vi "UI_main.vi"() -> ()   [LabVIEW 2013]
uses:
  parameter set for calibration.ctl
panel:
  in  "主要控制界面":enum32{"实时图像", "校准图样", "追踪数据", "设置"}(tab)
  out "力值估算":dbl
  out "往返测量":bool
  out "测量中":bool
  out "当前力值计算":dbl
  out "磁铁终点":dbl
  out "磁铁起点":dbl
  out "队列积压数据":u8(slide) scale=0.0..100.0
  out "测量模式":string
  out "文件存放路径":path
  out "测量进度":u8(slide) scale=0.0..100.0
  in  "当前温度":dbl
  in  "磁铁转数":dbl
  in  "磁铁位置":dbl
  in  "焦平面位置":dbl
  out "波形图":dbl[](graph)
  in  "校准磁球编号":dbl
  out "强度图":dbl[][](graph)
  out "D(Y)":dbl
  out "Y方向均值":dbl
  out "D(X)":dbl
  out "X方向均值":dbl
  out "Z_RMSE":dbl
  out "Z方向均值":dbl
  in  "参考磁球编号":enum16{""}(ring)
  in  "测量磁球编号":enum16{""}(ring)
  out "波形图表":dbl(graph)
  out "采样频率":dbl
  out "数据更新频率":dbl
  in  "旋转电机驱动":bool
  in  "步进电机驱动":bool
  in  "CCD相机驱动":bool
  out "单位像素大小":dbl
  in  "ROI size":enum16{"64 ", "128"}(ring)
  in  "显微镜放大倍数":dbl
  out "错误输出":errorcluster
  in  "错误输入（无错误）":errorcluster
  # "实验信息"
  # "数据监测"
  # "磁铁设置"
  # "驱动设置"
  # "ROI设置"
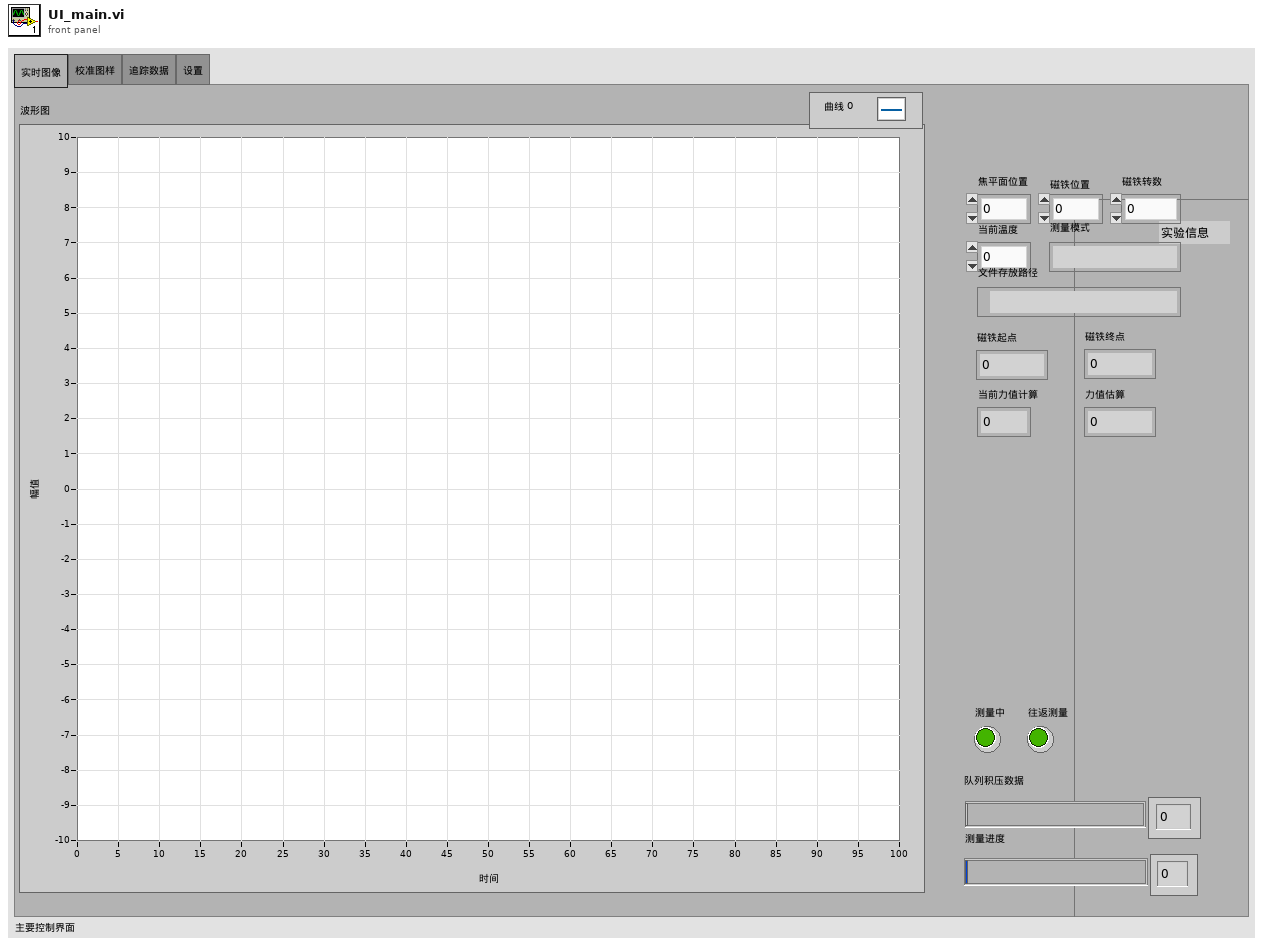
[diagram p1: front panel]
types:
  T1 = typedef "magnet_tweezers_命令.ctl" = enum16{"新建", "打开", "保存", "导出", "退出", "恢复初始设置", "校准", "测量Z值", "WLC", "相机驱动设置", "显微镜设置", "旋转电机设置", "平移电机设置", "保存参数设置", "参考磁球编号", "观测磁球编号", "修改磁铁位置", "修改磁铁转数", "修改当前温度", "修改焦平面位置", "修改磁球编号", "修改ROI大小", "修改显微镜放大倍数"}
  T2 = typedef "前面板命令.ctl" = cluster{"命令":T1, "数据":variant}
  T3 = typedef "tlc_Error Module Command Control.ctl" = enum16{"Initialize", "Handle Errors", "Report Errors"}
  T4 = typedef "parameter set for calibration.ctl" = cluster{"分子长度（bp）":i32, "磁球大小（直径）":dbl[unit], "校准起点":dbl, "校准步长":dbl, "每步采样数（frame）":i32, "首尾去除帧数(frame)":i32, "校准步数":i32, "底面位置":dbl, "R-step":sgl, "R-min":sgl, "R-max":sgl, "num":i32, "x_center":dbl, "y_center":dbl, "磁铁位置":dbl}
  T5 = typedef "parameter set for record.ctl" = cluster{"测量模式":enum16{"force ramp", "force jump", "force clamp"}, "测量起点":dbl, "数据存放路径":path, "加载率":dbl, "初始转数":dbl, "最终转数":dbl, "旋转速度":dbl, "松弛点":dbl, "绷紧点":dbl, "松弛时间":dbl, "绷紧时间":dbl, "步长":dbl, "总步数":dbl, "停留时间":dbl, "测量终点":dbl, "校准完毕？":bool}
  T6 = enum32{"invalid app kind", "Development System", "Run Time System", "Student Edition", "Embedded LabVIEW", "Evaluation", "Custom"}
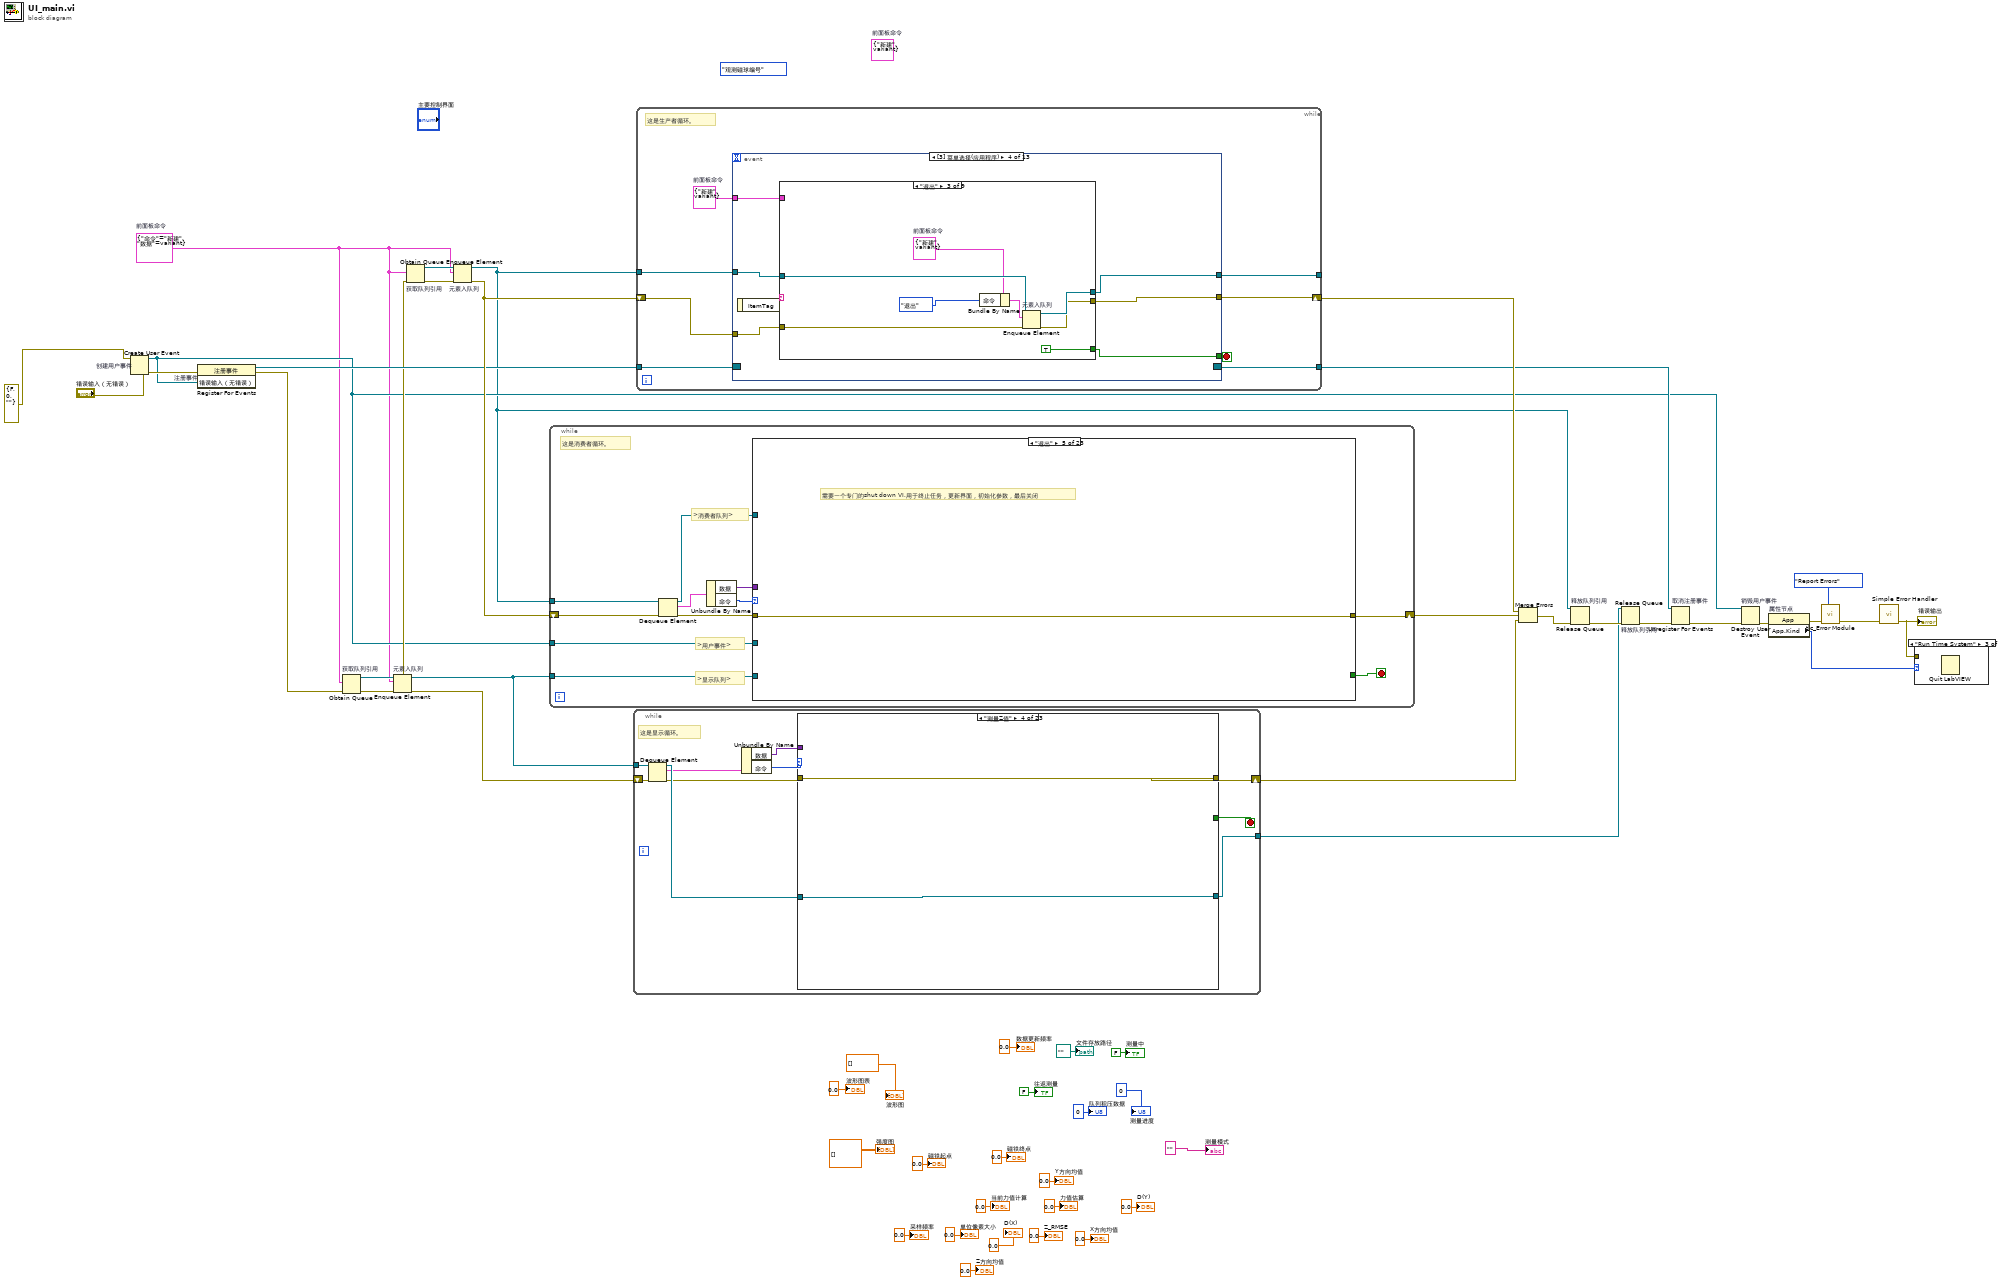
[diagram p0: block diagram]
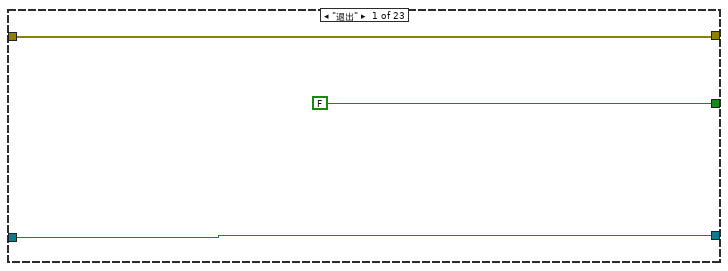
[diagram p8: hidden frame]
diagram:
  (unwired) magnet_tweezers_命令."观测磁球编号" ("命令")
  (unwired) T2 {"命令"=enum."新建", "数据"=variant}  # 前面板命令
  w24 = T2 {"命令"=enum."新建", "数据"=variant}  # 前面板命令
  n1 = Create User Event "创建用户事件"(user event datatype=errorcluster {"status"=FALSE, "code"=0, "source"=""} ("错误输入（无错误）"), error in="错误输入（无错误）") -> (user event=w34:refnum<user-event>, error out=w49:errorcluster)
  n2 = register-events "注册事件"(error in=w49, w34) -> (reference out=w48:refnum<event-registration>, error out=w39:errorcluster)  [unwired: 1 in]
  n3 = Obtain Queue "获取队列引用"(element data type=w24, error in (no error)=w39) -> (queue out=w40:refnum<queue>, error out=w41:errorcluster)  [unwired: 3 in, 1 out]
  n4 = Enqueue Element "元素入队列"(queue=w40, element=w24, error in (no error)=w41) -> (queue out=w33:refnum<queue>, error out=w38:errorcluster)  [unwired: 1 in, 1 out]
  n5 = Obtain Queue "获取队列引用"(element data type=w24, error in (no error)=w38) -> (queue out=w52:refnum<queue>, error out=w51:errorcluster)  [unwired: 3 in, 1 out]
  n6 = Enqueue Element "元素入队列"(queue=w52, element=w24, error in (no error)=w51) -> (queue out=w1:refnum<queue>, error out=w50:errorcluster)  [unwired: 1 in, 1 out]
  n7 = while {
    shift-right: [w53] -> w46
    shift-left: w50 -> [w61]
    tunnel: w1 -> [w63]
    tunnel: w34 -> [w56]
    tunnel: w33 -> [w55]
    stop <- w57 stop-if-true
    # ">显示队列>"
    # ">消费者队列>"
    # ">用户事件>"
    # "这是消费者循环。"
    n8 = Dequeue Element(queue=w63, error in (no error)=w61) -> (queue out=w62:refnum<queue>, element=w60:T2, error out=w58:errorcluster)  [unwired: 1 in, 1 out]
    n9 = Unbundle By Name(w60) -> ("数据"=w54:variant, "命令"=w59:T1)
    n10 = case shown="\"退出\"" w59 {
      tunnel: w62 -> [_ _ _ _ _ _ _ _ _ _ _ _ _ _ _ _ _ _ _ _ _ _ _]
      tunnel: w58 -> [w64 w66 w67 w68 w69 w70 w75 w79 w80 w81 w82 w83 w84 w85 w86 w87 w88 w89 w90 w91 w92 w93 w94]
      tunnel: [FALSE _ _ _ _ _ _ _ _ _ _ _ _ _ _ _ _ _ _ _ _ _ _] -> w57
      tunnel: w56 -> [_ _ _ _ _ _ _ _ _ _ _ _ _ _ _ _ _ _ _ _ _ _ _]
      tunnel: w55 -> [_ _ _ _ _ _ _ _ _ _ _ _ _ _ _ _ _ _ _ _ _ _ _]
      tunnel: w54 -> [_ _ _ _ _ _ w77 _ _ _ _ _ _ _ _ _ _ _ _ _ _ _ _]
      tunnel: [w64 w66 w67 w68 w69 w70 w71 w79 w80 w81 w82 w83 w84 w85 w86 w87 w88 w89 w90 w91 w92 w93 w94] -> w53
      frame "新建", Default {
      }
      frame "打开" {
      }
      frame "保存" {
      }
      frame "导出" {
      }
      frame "退出" {
        # "需要一个专门的shut down VI,用于终止任务，更新界面，初始化参数，最后关闭"
      }
      frame "恢复初始设置" {
      }
      frame "校准" {
        n11 = Variant To Data(error in=w75, type=T4 {"分子长度（bp）"=0, "磁球大小（直径）"=0.0, "校准起点"=0.0, "校准步长"=0.0, "每步采样数（frame）"=0, "首尾去除帧数(frame)"=0, "校准步数"=0, "底面位置"=0.0, "R-step"=1.0, "R-min"=0.0, "R-max"=0.0, "num"=2, "x_center"=0.0, "y_center"=0.0, "磁铁位置"=0.0} ("parameter for calibration"), Variant=w77) -> (data=w72:T4, error out=w73:errorcluster)
        n12 = Unbundle By Name(w72) -> ("校准步数"=w74:i32)
        n13 = for {
          N: w74 -> [_]
          tunnel: w73 -> [w78]
          shift-right: [w78] -> w71
          shift-left: _ -> [_]
          tunnel: w72 -> [_]
        }
      }
      frame "测量Z值" {
      }
      frame "WLC" {
      }
      frame "相机驱动设置" {
      }
      frame "显微镜设置" {
      }
      frame "旋转电机设置" {
      }
      frame "平移电机设置" {
      }
      frame "保存参数设置" {
      }
      frame "参考磁球编号" {
      }
      frame "观测磁球编号" {
      }
      frame "修改磁铁位置" {
      }
      frame "修改磁铁转数" {
      }
      frame "修改当前温度" {
      }
      frame "修改焦平面位置" {
      }
      frame "修改磁球编号" {
      }
      frame "修改ROI大小" {
      }
      frame "修改显微镜放大倍数" {
      }
    }
  }
  n14 = while {
    shift-right: [w100] -> w32
    shift-left: w38 -> [w102]
    tunnel: [w103] -> w35
    tunnel: w33 -> [w98]
    stop <- w99 stop-if-true
    # "这是显示循环。"
    n15 = Dequeue Element(queue=w98, error in (no error)=w102) -> (queue out=w104:refnum<queue>, element=w96:T2, error out=w101:errorcluster)  [unwired: 1 in, 1 out]
    n16 = Unbundle By Name(w96) -> ("数据"=w95:variant, "命令"=w97:T1)
    n17 = case shown="\"测量Z值\"" w97 {
      tunnel: w104 -> [w107 w109 w111 w113 w115 w117 w119 w121 w123 w125 w127 w129 w131 w133 w135 w137 w139 w141 w143 w145 w147 w149 w151]
      tunnel: [w107 w109 w111 w113 w115 w117 w119 w121 w123 w125 w127 w129 w131 w133 w135 w137 w139 w141 w143 w145 w147 w149 w151] -> w103
      tunnel: w101 -> [w105 w108 w110 w112 w114 w116 w118 w120 w122 w124 w126 w128 w130 w132 w134 w136 w138 w140 w142 w144 w146 w148 w150]
      tunnel: [w105 w108 w110 w112 w114 w116 w118 w120 w122 w124 w126 w128 w130 w132 w134 w136 w138 w140 w142 w144 w146 w148 w150] -> w100
      tunnel: [FALSE _ _ _ _ _ _ _ _ _ _ _ _ _ _ _ _ _ _ _ _ _ _] -> w99
      tunnel: w95 -> [_ _ _ _ _ _ _ _ _ _ _ _ _ _ _ _ _ _ _ _ _ _ _]
      frame "退出" {
      }
      frame "恢复初始设置" {
      }
      frame "校准" {
      }
      frame "测量Z值" {
      }
      frame "WLC" {
      }
      frame "相机驱动设置" {
      }
      frame "显微镜设置" {
      }
      frame "旋转电机设置" {
      }
      frame "平移电机设置" {
      }
      frame "保存参数设置" {
      }
      frame "参考磁球编号" {
      }
      frame "观测磁球编号" {
      }
      frame "修改磁铁位置" {
      }
      frame "修改磁铁转数" {
      }
      frame "修改当前温度" {
      }
      frame "修改焦平面位置" {
      }
      frame "修改磁球编号" {
      }
      frame "修改ROI大小" {
      }
      frame "修改显微镜放大倍数" {
      }
      frame "导出" {
      }
      frame "保存" {
      }
      frame "打开" {
      }
      frame "新建" {
      }
    }
  }
  n18 = while {
    shift-right: [w157] -> w45
    shift-left: w50 -> [w158]
    tunnel: w48 -> [w154]
    tunnel: [w153] -> w43
    tunnel: w1 -> [w159]
    tunnel: [w155] -> _
    stop <- w156 stop-if-true
    w152 = T2 {"命令"=enum."新建", "数据"=variant}  # 前面板命令
    # "这是生产者循环。"
    n19 = event shown="[3] 菜单选择(应用程序)" {
      selector: w154 -> [_ _ _ _ _ _ _ _ _ _ _ _ _]
      dyn-events: [_ _ _ _ _ _ _ _ _ _ _ _ _] -> w153
      timeout: _ -> [_ _ _ _ _ _ _ _ _ _ _ _ _]
      tunnel: w159 -> [w168 w175 w185 w196 w332 w342 w351 w360 w369 w378 w387 w396 w405]
      tunnel: w158 -> [w167 w173 w184 w195 w330 w340 w349 w358 w367 w376 w385 w394 w403]
      tunnel: [w166 w171 w183 w193 w329 w339 w348 w357 w366 w375 w384 w393 w402] -> w157
      tunnel: [FALSE FALSE FALSE w192 _ _ _ _ _ _ _ _ _] -> w156
      tunnel: [w165 w174 w182 w194 w331 w341 w350 w359 w368 w377 w386 w395 w404] -> w155
      tunnel: w152 -> [w164 w178 w186 w190 w333 w343 w352 w361 w370 w379 w388 w397 w406]
      event "磁铁位置": Value Change {
        n20 = event-data() -> ()  [unwired: 1 in, 1 out]
        n21 = To Variant(anything="磁铁位置") -> (Variant=w163:variant)
        n22 = Bundle By Name(cluster=w164, "命令"=magnet_tweezers_命令."修改磁铁位置", "数据"=w163) -> (w161:T2)
        n23 = Enqueue Element(queue=w168, element=w161, error in (no error)=w167) -> (queue out=w165:refnum<queue>, error out=w166:errorcluster)  [unwired: 1 in, 1 out]
      }
      event "测量磁球编号": Value Change {
        # "从用户端获得一个队列，将情境发送至消费者循环。"
        n24 = event-data() -> ()  [unwired: 1 in, 2 out]
        n25 = To Variant(anything="测量磁球编号") -> (Variant=w176:variant)
        n26 = Bundle By Name(cluster=w178, "命令"=magnet_tweezers_命令."观测磁球编号", "数据"=w176) -> (w172:T2)
        n27 = Enqueue Element "元素入队列"(queue=w175, element=w172, error in (no error)=w173) -> (queue out=w174:refnum<queue>, error out=w171:errorcluster)  [unwired: 1 in, 1 out]
      }
      event "参考磁球编号": Value Change {
        n28 = event-data() -> ()  [unwired: 1 in, 1 out]
        n29 = To Variant(anything="参考磁球编号") -> (Variant=w188:variant)
        n30 = Bundle By Name(cluster=w186, "命令"=magnet_tweezers_命令."参考磁球编号", "数据"=w188) -> (w187:T2)
        n31 = Enqueue Element "元素入队列"(queue=w185, element=w187, error in (no error)=w184) -> (queue out=w182:refnum<queue>, error out=w183:errorcluster)  [unwired: 1 in, 1 out]
      }
      event Menu Selection (App) {
        n32 = event-data() -> ("ItemTag"=w191:string)  [unwired: 1 in]
        n33 = case shown="\"退出\"" w191 {
          tunnel: w196 -> [w197 w219 w248 w251 w259 w265 w288 w305 w322]
          tunnel: w195 -> [w205 w227 w246 w250 w257 w264 w283 w304 w321]
          tunnel: [w201 w223 w247 w251 w258 w263 w287 w303 w324] -> w194
          tunnel: [w202 w224 w245 w250 w256 w262 w286 w302 w323] -> w193
          tunnel: [FALSE FALSE TRUE FALSE FALSE FALSE FALSE FALSE FALSE] -> w192
          tunnel: w190 -> [_ _ _ _ w254 w260 w284 w300 w327]
          frame "保存" {
            n34 = call "File Dialog"("error in"=w205) -> ("selected path"=w198:path, "exists"=w204:bool, "cancelled"=w203:bool, "error out"=w200:errorcluster)  [unwired: 11 in]
            n35 = Compound Arithmetic op=OR(w204, invert w203) -> (w199:bool)
            n36 = case shown="真" w199 {
              tunnel: [w209 w218] -> w202
              tunnel: [w207 w217] -> w201
              tunnel: w200 -> [w210 w216]
              tunnel: w198 -> [_ w215]
              tunnel: w197 -> [w207 w213]
              frame False {
                n37 = call "Clear Specific Error.vi"("错误输入（无错误）"=w210, "代码"=43 ("Code")) -> ("错误输出"=w209:errorcluster)  [unwired: 5 in]
              }
              frame True {
                w212 = T2 {"命令"=enum."新建", "数据"=variant}  # 前面板命令
                n38 = To Variant(anything=w215) -> (Variant=w214:variant)
                n39 = Bundle By Name(cluster=w212, "数据"=w214) -> (w211:T2)
                n40 = Enqueue Element(queue=w213, element=w211, error in (no error)=w216) -> (queue out=w217:refnum<queue>, error out=w218:errorcluster)  [unwired: 1 in, 1 out]
              }
            }
          }
          frame "打开" {
            n41 = call "File Dialog2"("error in"=w227) -> ("selected path"=w220:path, "exists"=w226:bool, "cancelled"=w225:bool, "error out"=w222:errorcluster)  [unwired: 11 in]
            n42 = Compound Arithmetic op=OR(w226, invert w225) -> (w221:bool)
            n43 = case shown="真" w221 {
              tunnel: [w231 w240] -> w224
              tunnel: [w229 w239] -> w223
              tunnel: w222 -> [w232 w238]
              tunnel: w220 -> [_ w237]
              tunnel: w219 -> [w229 w235]
              frame False {
                n44 = call "Clear Specific Error.vi"("错误输入（无错误）"=w232, "代码"=43 ("Code")) -> ("错误输出"=w231:errorcluster)  [unwired: 5 in]
              }
              frame True {
                w234 = T2 {"命令"=enum."新建", "数据"=variant}  # 前面板命令
                n45 = To Variant(anything=w237) -> (Variant=w236:variant)
                n46 = Bundle By Name(cluster=w234, "数据"=w236) -> (w233:T2)
                n47 = Enqueue Element(queue=w235, element=w233, error in (no error)=w238) -> (queue out=w239:refnum<queue>, error out=w240:errorcluster)  [unwired: 1 in, 1 out]
              }
            }
          }
          frame "退出" {
            w243 = T2 {"命令"=enum."新建", "数据"=variant}  # 前面板命令
            n48 = Bundle By Name(cluster=w243, "命令"=magnet_tweezers_命令."退出") -> (w242:T2)
            n49 = Enqueue Element "元素入队列"(queue=w248, element=w242, error in (no error)=w246) -> (queue out=w247:refnum<queue>, error out=w245:errorcluster)  [unwired: 1 in, 1 out]
          }
          frame "新建 ", Default {
          }
          frame "恢复初始设置" {
            n50 = Bundle By Name(cluster=w254, "命令"=magnet_tweezers_命令."恢复初始设置") -> (w253:T2)
            n51 = Enqueue Element "元素入队列"(queue=w259, element=w253, error in (no error)=w257) -> (queue out=w258:refnum<queue>, error out=w256:errorcluster)  [unwired: 1 in, 1 out]
          }
          frame "保存参数设置" {
            n52 = call "dialog_box for record.vi"("错误输入（无错误）"=w264) -> ("错误输出"=w268:errorcluster, "参数输出"=w267:T5, "Cancelled?"=w266:bool)  [unwired: 7 in, 1 out]
            n53 = case shown="假" w266 {
              tunnel: w265 -> [w277 w279]
              tunnel: w268 -> [w276 w278]
              tunnel: [w275 w278] -> w262
              tunnel: [w274 w279] -> w263
              tunnel: w267 -> [w273 _]
              tunnel: w260 -> [w270 _]
              frame False {
                n54 = To Variant(anything=w273) -> (Variant=w272:variant)
                n55 = Bundle By Name(cluster=w270, "命令"=magnet_tweezers_命令."保存参数设置", "数据"=w272) -> (w271:T2)
                n56 = Enqueue Element "元素入队列"(queue=w277, element=w271, error in (no error)=w276) -> (queue out=w274:refnum<queue>, error out=w275:errorcluster)  [unwired: 1 in, 1 out]
              }
              frame True {
              }
            }
          }
          frame "校准" {
            n57 = call "dialog_box for calibration.vi"("error in (no error)"=w283) -> ("error out"=w282:errorcluster, "parameter for calibration out"=w281:T4, "Cancelled?"=w280:bool)  [unwired: 8 in]
            n58 = case shown="假" w280 {
              tunnel: w288 -> [w297 w299]
              tunnel: w282 -> [w296 w298]
              tunnel: [w295 w298] -> w286
              tunnel: [w294 w299] -> w287
              tunnel: w284 -> [w291 _]
              tunnel: w281 -> [w289 _]
              frame False {
                n59 = To Variant(anything=w289) -> (Variant=w293:variant)
                n60 = Bundle By Name(cluster=w291, "命令"=magnet_tweezers_命令."观测磁球编号", "数据"=w293) -> (w292:T2)
                n61 = Enqueue Element "元素入队列"(queue=w297, element=w292, error in (no error)=w296) -> (queue out=w294:refnum<queue>, error out=w295:errorcluster)  [unwired: 1 in, 1 out]
              }
              frame True {
              }
            }
          }
          frame "测量Z值" {
            n62 = call "dialog_box for record.vi"("错误输入（无错误）"=w304) -> ("错误输出"=w306:errorcluster, "参数输出"=w307:T5, "Cancelled?"=w308:bool)  [unwired: 7 in, 1 out]
            n63 = case shown="假" w308 {
              tunnel: w305 -> [w317 w319]
              tunnel: w306 -> [w316 w318]
              tunnel: [w315 w318] -> w302
              tunnel: [w314 w319] -> w303
              tunnel: w307 -> [w313 _]
              tunnel: w300 -> [w310 _]
              frame False {
                n64 = To Variant(anything=w313) -> (Variant=w312:variant)
                n65 = Bundle By Name(cluster=w310, "命令"=magnet_tweezers_命令."测量Z值", "数据"=w312) -> (w311:T2)
                n66 = Enqueue Element "元素入队列"(queue=w317, element=w311, error in (no error)=w316) -> (queue out=w314:refnum<queue>, error out=w315:errorcluster)  [unwired: 1 in, 1 out]
              }
              frame True {
              }
            }
          }
          frame "WLC" {
            n67 = Bundle By Name(cluster=w327, "命令"=magnet_tweezers_命令."WLC") -> (w325:T2)
            n68 = Enqueue Element "元素入队列"(queue=w322, element=w325, error in (no error)=w321) -> (queue out=w324:refnum<queue>, error out=w323:errorcluster)  [unwired: 1 in, 1 out]
          }
        }
      }
      event "磁铁转数": Value Change {
        n69 = event-data() -> ()  [unwired: 1 in, 2 out]
        n70 = To Variant(anything="磁铁转数") -> (Variant=w336:variant)
        n71 = Bundle By Name(cluster=w333, "命令"=magnet_tweezers_命令."修改磁铁转数", "数据"=w336) -> (w335:T2)
        n72 = Enqueue Element(queue=w332, element=w335, error in (no error)=w330) -> (queue out=w331:refnum<queue>, error out=w329:errorcluster)  [unwired: 1 in, 1 out]
      }
      event "当前温度": Value Change {
        n73 = event-data() -> ()  [unwired: 1 in, 2 out]
        n74 = To Variant(anything="当前温度") -> (Variant=w345:variant)
        n75 = Bundle By Name(cluster=w343, "命令"=magnet_tweezers_命令."修改当前温度", "数据"=w345) -> (w344:T2)
        n76 = Enqueue Element(queue=w342, element=w344, error in (no error)=w340) -> (queue out=w341:refnum<queue>, error out=w339:errorcluster)  [unwired: 1 in, 1 out]
      }
      event "焦平面位置": Value Change {
        n77 = event-data() -> ()  [unwired: 1 in, 2 out]
        n78 = To Variant(anything="焦平面位置") -> (Variant=w354:variant)
        n79 = Bundle By Name(cluster=w352, "命令"=magnet_tweezers_命令."修改焦平面位置", "数据"=w354) -> (w353:T2)
        n80 = Enqueue Element(queue=w351, element=w353, error in (no error)=w349) -> (queue out=w350:refnum<queue>, error out=w348:errorcluster)  [unwired: 1 in, 1 out]
      }
      event "校准磁球编号": Value Change {
        n81 = event-data() -> ()  [unwired: 1 in, 2 out]
        n82 = To Variant(anything="校准磁球编号") -> (Variant=w363:variant)
        n83 = Bundle By Name(cluster=w361, "命令"=magnet_tweezers_命令."修改磁球编号", "数据"=w363) -> (w362:T2)
        n84 = Enqueue Element(queue=w360, element=w362, error in (no error)=w358) -> (queue out=w359:refnum<queue>, error out=w357:errorcluster)  [unwired: 1 in, 1 out]
      }
      event "ROI size": Value Change {
        n85 = event-data() -> ()  [unwired: 1 in, 2 out]
        n86 = To Variant(anything="ROI size") -> (Variant=w372:variant)
        n87 = Bundle By Name(cluster=w370, "命令"=magnet_tweezers_命令."修改ROI大小", "数据"=w372) -> (w371:T2)
        n88 = Enqueue Element(queue=w369, element=w371, error in (no error)=w367) -> (queue out=w368:refnum<queue>, error out=w366:errorcluster)  [unwired: 1 in, 1 out]
      }
      event "显微镜放大倍数": Value Change {
        n89 = event-data() -> ()  [unwired: 1 in, 2 out]
        n90 = To Variant(anything="显微镜放大倍数") -> (Variant=w381:variant)
        n91 = Bundle By Name(cluster=w379, "命令"=magnet_tweezers_命令."修改显微镜放大倍数", "数据"=w381) -> (w380:T2)
        n92 = Enqueue Element(queue=w378, element=w380, error in (no error)=w376) -> (queue out=w377:refnum<queue>, error out=w375:errorcluster)  [unwired: 1 in, 1 out]
      }
      event "CCD相机驱动": Value Change {
        n93 = event-data() -> ()  [unwired: 1 in, 2 out]
        n94 = To Variant(anything="CCD相机驱动") -> (Variant=w390:variant)
        n95 = Bundle By Name(cluster=w388, "命令"=magnet_tweezers_命令."相机驱动设置", "数据"=w390) -> (w389:T2)
        n96 = Enqueue Element(queue=w387, element=w389, error in (no error)=w385) -> (queue out=w386:refnum<queue>, error out=w384:errorcluster)  [unwired: 1 in, 1 out]
      }
      event "步进电机驱动": Value Change {
        n97 = event-data() -> ()  [unwired: 1 in, 2 out]
        n98 = To Variant(anything="步进电机驱动") -> (Variant=w399:variant)
        n99 = Bundle By Name(cluster=w397, "命令"=magnet_tweezers_命令."平移电机设置", "数据"=w399) -> (w398:T2)
        n100 = Enqueue Element(queue=w396, element=w398, error in (no error)=w394) -> (queue out=w395:refnum<queue>, error out=w393:errorcluster)  [unwired: 1 in, 1 out]
      }
      event "旋转电机驱动": Value Change {
        n101 = event-data() -> ()  [unwired: 1 in, 2 out]
        n102 = To Variant(anything="旋转电机驱动") -> (Variant=w408:variant)
        n103 = Bundle By Name(cluster=w406, "命令"=magnet_tweezers_命令."旋转电机设置", "数据"=w408) -> (w407:T2)
        n104 = Enqueue Element(queue=w405, element=w407, error in (no error)=w403) -> (queue out=w404:refnum<queue>, error out=w402:errorcluster)  [unwired: 1 in, 1 out]
      }
    }
  }
  n105 = Merge Errors(w45, w46, w32) -> (w44:errorcluster)
  n106 = Release Queue "释放队列引用"(queue=w1, error in (no error)=w44) -> (error out=w37:errorcluster)  [unwired: 1 in, 2 out]
  n107 = Release Queue "释放队列引用"(queue=w35, error in (no error)=w37) -> (error out=w36:errorcluster)  [unwired: 1 in, 2 out]
  n108 = Unregister For Events "取消注册事件"(event registration refnum=w43, error in=w36) -> (error out=w42:errorcluster)
  n109 = Destroy User Event "销毁用户事件"(user event=w34, error in=w42) -> (error out=w27:errorcluster)
  n110 = property on="属性节点" class="App"(error in=w27) -> (error out=w29:errorcluster, "App.Kind"=w28:T6)  [unwired: 1 in, 1 out]
  n111 = call "tlc_Error Module.vi"("命令（处理错误）"=tlc_Error_Module_Command_Control."Report Errors" ("Command (Handle Errors"), "错误输入（无错误）"=w29) -> ("错误输出"=w30:errorcluster)  [unwired: 8 in, 1 out]
  n112 = call <vilib>:"Simple Error Handler.vi"("error in (no error)"=w30) -> ("error out"=w26:errorcluster)  [unwired: 4 in, 4 out]
  "错误输出" <- w26
  n113 = case shown="\"Run Time System\"" w28 {
    tunnel: w26 -> [_ _ _ _ _ _ _]
    frame "invalid app kind", Default {
    }
    frame "Development System" {
    }
    frame "Run Time System" {
      n114 = Quit LabVIEW() -> ()  [unwired: 1 in]
    }
    frame "Student Edition" {
    }
    frame "Embedded LabVIEW" {
    }
    frame "Evaluation" {
    }
    frame "Custom" {
    }
  }
  "波形图" <- dbl[] [] ("波形图")
  "强度图" <- dbl[][] [] ("强度图")
  "波形图表" <- 0.0 ("波形图表")
  "测量模式" <- "" ("测量模式")
  "文件存放路径" <- path "" ("文件存放路径")
  "采样频率" <- 0.0 ("采样频率")
  "Z_RMSE" <- 0.0 ("Z_RMSE")
  "X方向均值" <- 0.0 ("X方向均值")
  "D(X)" <- 0.0 ("D(X)")
  "当前力值计算" <- 0.0 ("当前力值计算")
  "力值估算" <- 0.0 ("力值估算")
  "数据更新频率" <- 0.0 ("数据更新频率")
  "Z方向均值" <- 0.0 ("Z方向均值")
  "测量中" <- FALSE ("测量中")
  "往返测量" <- FALSE ("往返测量")
  "Y方向均值" <- 0.0 ("Y方向均值")
  "队列积压数据" <- u8 0 ("队列积压数据")
  "D(Y)" <- 0.0 ("D(Y)")
  "测量进度" <- u8 0 ("测量进度")
  "单位像素大小" <- 0.0 ("单位像素大小")
  "磁铁起点" <- 0.0 ("磁铁起点")
  "磁铁终点" <- 0.0 ("磁铁终点")
